vi "calculatorProgram.vi"() -> ()   [LabVIEW 2021]
panel:
  out "Calculated Value":dbl
  in  "Number2":dbl
  in  "Number1":dbl
  in  "Cases":T1(ring)
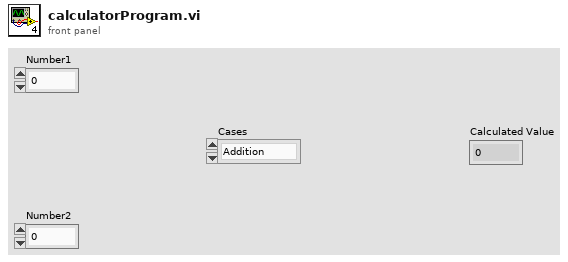
[diagram p1: front panel]
types:
  T1 = enum16{"Addition", "Subtraction", "Prduct", "Division", "Square", "Square Root"}
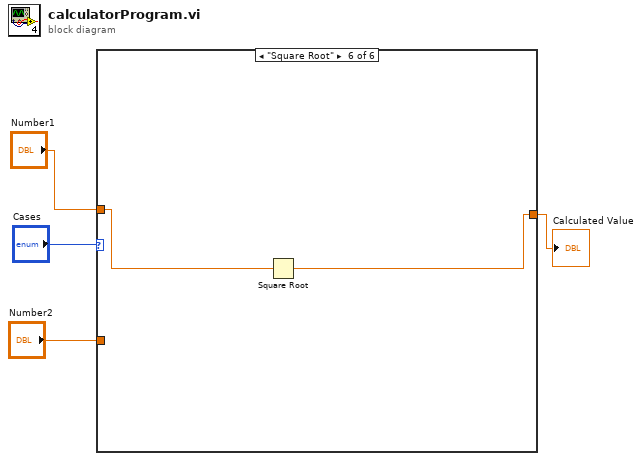
[diagram p0: block diagram]
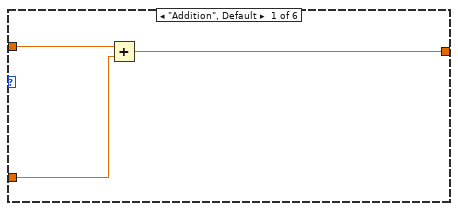
[diagram p2: hidden frame]
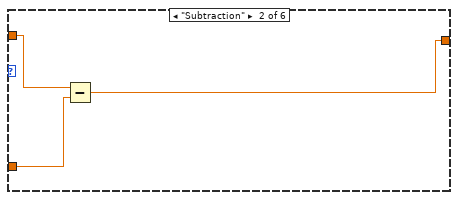
[diagram p3: hidden frame]
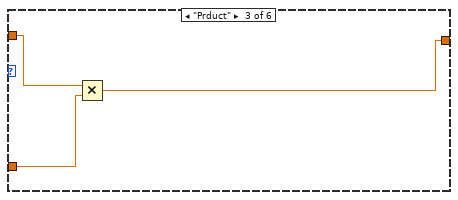
[diagram p4: hidden frame]
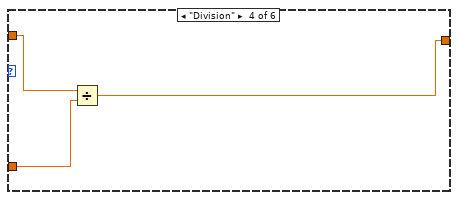
[diagram p5: hidden frame]
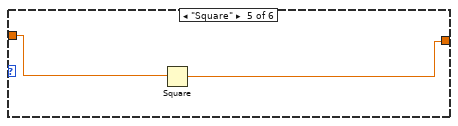
[diagram p6: hidden frame]
diagram:
  n1 = case shown="\"Square Root\"" "Cases" {
    tunnel: "Number1" -> [w7 w10 w13 w16 w18 w20]
    tunnel: "Number2" -> [w6 w9 w12 w15 _ _]
    tunnel: [w5 w8 w11 w14 w17 w19] -> w2
    frame "Addition", Default {
      n2 = Add(x=w7, y=w6) -> (x+y=w5:dbl)
    }
    frame "Subtraction" {
      n3 = Subtract(x=w10, y=w9) -> (x-y=w8:dbl)
    }
    frame "Prduct" {
      n4 = Multiply(x=w13, y=w12) -> (x*y=w11:dbl)
    }
    frame "Division" {
      n5 = Divide(x=w16, y=w15) -> (x/y=w14:dbl)
    }
    frame "Square" {
      n6 = Square(x=w18) -> (x^2=w17:dbl)
    }
    frame "Square Root" {
      n7 = Square Root(x=w20) -> (sqrt(x)=w19:dbl)
    }
  }
  "Calculated Value" <- w2
